vi "S8300E_CheckSN_Manual.vi"() -> ()   [LabVIEW 2011]
panel:
  out "UUT SN":string
  out "UUT MAC List":string
  out "CMD-LIST":cluster{string, string, string, string}[](array[cluster])
  out "log msg":string
  out "VISA resource name out":refnum<visa-resource-name>
  out "BEGIN TIME":u32
  out "進行狀況":string
  # "Error Code:SN-BIOS\nError Code:SN-DMI"
  # "S8300E Program SN (接UART COM9)"
  # "2014-12-12"
  # "Step1:Get Serial Number from BIOS Flash\nStep2:Get Serial Number from DMI table"
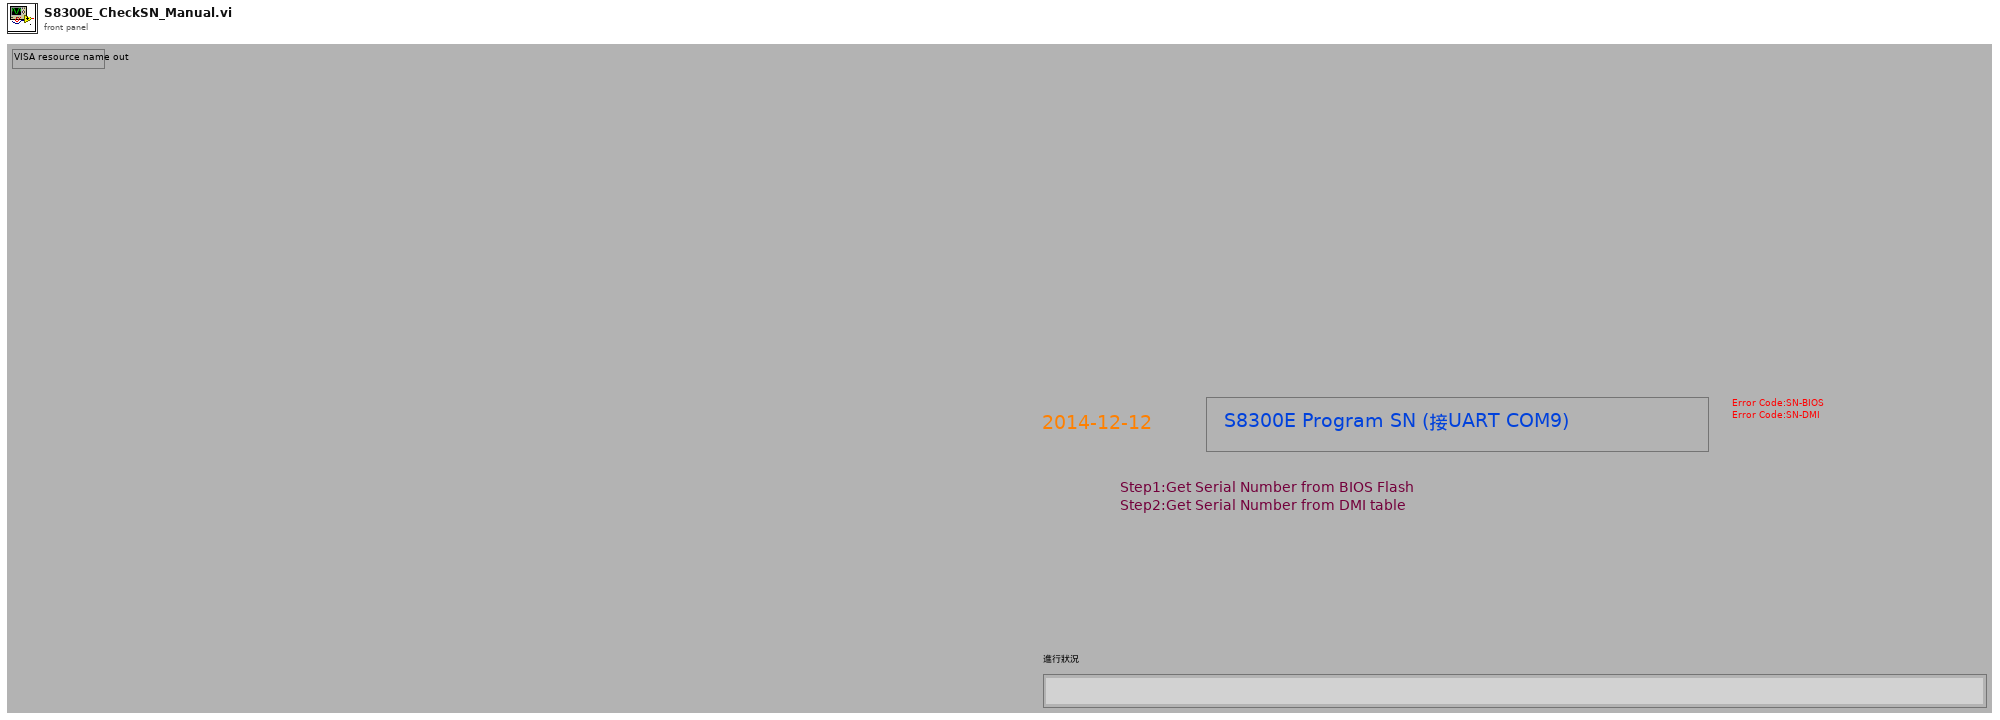
[diagram p1: front panel]
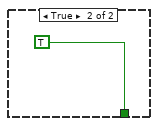
[diagram p7: hidden frame]
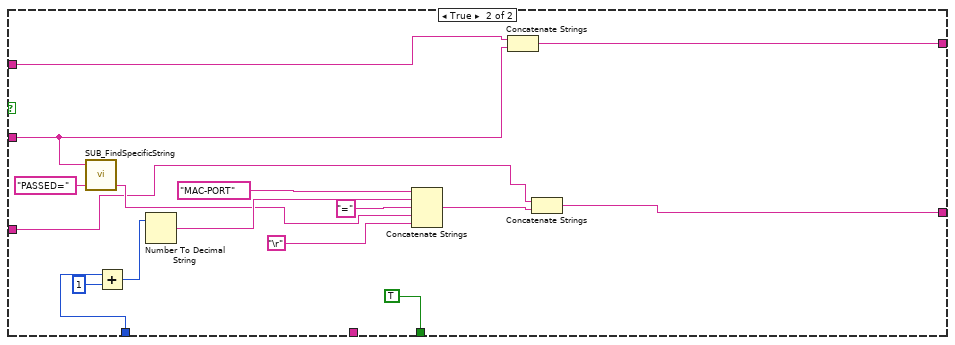
[diagram p9: hidden frame]
diagram:
  n1 = flat-sequence {
    frame #0 {
      n2 = Tick Count (ms)() -> (millisecond timer value=→"BEGIN TIME":u32)
    }
    frame #1 {
      n3 = property on="進行狀況" class="Str"("Blinking"=TRUE) -> ()  [unwired: 2 in, 2 out]
      "進行狀況" <- "進入測試準備中...." ("進行狀況")
      "UUT SN" <- ""
    }
    frame #2 {
      n4 = call "SUB_SearchFile_inFolder.vi"("Search Filename in Folder"="S8300E_sfcs_misc.txt") -> ("File Existing True/Flase"=w5:bool)  [unwired: 1 in]
      n5 = case shown="False" w5 {
        frame False {
          n6 = flat-sequence {
            frame #0 {
              n7 = call "Display Message to User"() -> ()  [unwired: 10 in, 2 out]
            }
            frame #1 {
              n8 = call "SUB_Writelog.vi"("Pass/Fail"="Fail:S8300E_CheckSN_Manual") -> ()  [unwired: 2 in]
            }
            frame #2 {
              n9 = Quit LabVIEW(quit? (T)=TRUE) -> ()
            }
          }
        }
        frame True {
        }
      }
    }
    frame #3 {
      n10 = call "Prompt User for Input"() -> ("待測物條碼序號"=w9:string)  [unwired: 17 in, 2 out]
      n11 = local write "UUT SN"(w9) -> ()
    }
    frame #4 {
      n12 = local read "UUT SN"() -> (w11:string)
      n13 = Concatenate Strings("PASSED=", w11) -> (w10:string)
      n14 = Concatenate Strings("PASSED=", w11) -> (w13:string)
      n15 = Concatenate Strings("./ser.sh -w -f  ", w11, "\r") -> (w32:string)
      n16 = Concatenate Strings("./ser.sh -r -f  ", "\r") -> (w28:string)
      n17 = Concatenate Strings("./ser.sh -r -d ", "\r") -> (w25:string)
      n18 = Bundle(w32, "PASSED=", "Set Serial Number to BIOS Flash", "SN-BIOS") -> ()  [unwired: 1 in, 1 out]
      n19 = Bundle(w28, w13, "Get Serial Number from BIOS Flash", "SN-BIOS") -> (w20:cluster{string, string, string, string})  [unwired: 1 in]
      n20 = Bundle(w25, w10, "Get Serial Number from DMI table", "SN-DMI") -> (w19:cluster{string, string, string, string})  [unwired: 1 in]
      n21 = Build Array(w20, w19) -> (→"CMD-LIST":cluster{string, string, string, string}[])
    }
    frame #5 {
      n22 = case shown="True" TRUE {
        frame False {
        }
        frame True {
          n23 = call "SUB_COM1_CLOSE.vi"("VISA resource name"=refnum<visa-resource-name> "COM9") -> ()  [unwired: 3 in]
        }
      }
    }
    frame #6 {
      n24 = case shown="True" TRUE {
        frame False {
        }
        frame True {
          n25 = call "SUB_COM9_INIT.vi"("baud rate"=u32 115200) -> ("VISA resource name out"=w40:refnum<visa-resource-name>)  [unwired: 1 in, 1 out]
          "VISA resource name out" <- w40
          n26 = call "SUB_COM1Wrt.vi"("VISA resource name"=w40, "write buffer"="\r") -> ("duplicate VISA resource name"=w37:refnum<visa-resource-name>)  [unwired: 1 in, 1 out]
          n27 = call "SUB_ContinueCom1Read.vi"("Numeric"=1200, "duplicate VISA resource name 2"=w37) -> ()  [unwired: 1 in, 3 out]
        }
      }
    }
    frame #7 {
      n28 = case shown="True" TRUE {
        frame False {
        }
        frame True {
          n29 = while {
            stop <- w52 stop-if-true
            w43 = "\r"
            n30 = Concatenate Strings(w43, w43, w43) -> (w44:string)
            n31 = local read "VISA resource name out"() -> (w45:refnum<visa-resource-name>)
            n32 = call "SUB_COM1Wrt.vi"("VISA resource name"=w45, "write buffer"=w44) -> ("duplicate VISA resource name"=w51:refnum<visa-resource-name>)  [unwired: 1 in, 1 out]
            n33 = Tick Count (ms)() -> (millisecond timer value=w50:u32)
            n34 = call "SUB_READ_COM1_FindString_timeout.vi"("Find this String"="s8300e_func_test#", "Timeout Seccond"=3.0, "Begin time"=w50, "duplicate VISA resource name 2"=w51) -> ("Output String"=w46:string, "Found String"=w47:bool)  [unwired: 1 in, 1 out]
            n35 = case shown="False" w47 {
              tunnel: [w54 TRUE] -> w52
              tunnel: w46 -> [w53 _]
              frame False {
                n36 = call "SUB_YESNO.vi"("Debug View"=w53, "Status"="UART無正確反應!需有S8300E字串") -> ("yes/no"=w57:enum32{"No Selection", "Yes", "No", "None"})  [unwired: 1 in]
                n37 = Equal?(x=w57, y=enum32{"No Selection", "Yes", "No", "None"}."No") -> (x = y?=w55:bool)
                n38 = case shown="True" w55 {
                  tunnel: [_ w59] -> w54
                  frame False {
                  }
                  frame True {
                    n39 = flat-sequence {
                      tunnel: [w63] -> w59
                      frame #0 {
                        n40 = call "SUB_Writelog.vi"("Pass/Fail"="Fail:S8300E_CheckSN_Manual") -> ()  [unwired: 2 in]
                      }
                      frame #1 {
                        n41 = call "SUB_SFCS_SendResult.vi"("ErrorCode"="UART", "PASS_Fail (1/0)"=i8 0) -> ()  [unwired: 1 out]
                      }
                      frame #2 {
                        w63 = TRUE ("quit? (T)")
                        n42 = Quit LabVIEW(quit? (T)=w63) -> ()
                      }
                    }
                  }
                }
              }
              frame True {
              }
            }
          }
        }
      }
    }
    frame #8 {
      n43 = local read "CMD-LIST"() -> (w67:cluster{string, string, string, string}[])
      n44 = Array Size(array=w67) -> (size(s)=w70:i32)
      n45 = for {
        N: w70 -> [_]
        shift-right: [w75] -> w68
        shift-left: "" -> [w74]
        shift-right: [w72] -> w65
        shift-left: "" -> [w71]
        i -> [w73]
        n46 = while {
          tunnel: w73 -> [w94]
          tunnel: [w86] -> w75
          tunnel: w74 -> [w85]
          tunnel: w73 -> [w78]
          tunnel: [w77] -> w72
          tunnel: w71 -> [w76]
          stop <- w88 stop-if-true
          n47 = local read "VISA resource name out"() -> (w90:refnum<visa-resource-name>)
          n48 = local read "CMD-LIST"() -> (w84:cluster{string, string, string, string}[])
          n49 = Index Array(array=w84, index=w94) -> (element=w83:cluster{string, string, string, string})
          n50 = Unbundle(w83) -> (w82:string, w80:string, w81:string, w79:string)
          n51 = call "SUB_COM1Wrt.vi"("VISA resource name"=w90, "write buffer"=w82) -> ("duplicate VISA resource name"=w93:refnum<visa-resource-name>)  [unwired: 1 in, 1 out]
          n52 = Tick Count (ms)() -> (millisecond timer value=w92:u32)
          n53 = call "SUB_READ_COM1_FindString_timeout.vi"("Find this String"=w80, "Timeout Seccond"=2.0, "Begin time"=w92, "duplicate VISA resource name 2"=w93) -> ("Output String"=w87:string, "Found String"=w89:bool)  [unwired: 1 in, 1 out]
          n54 = local write "進行狀況"(w81) -> ()
          n55 = case shown="False" w89 {
            tunnel: [_ TRUE] -> w88
            tunnel: w87 -> [w105 w122]
            tunnel: [w101 w127] -> w86
            tunnel: w85 -> [w101 w126]
            tunnel: w79 -> [w100 _]
            tunnel: w78 -> [_ w118]
            tunnel: [w95 w114] -> w77
            tunnel: w76 -> [w95 w113]
            frame False {
              n56 = local read "進行狀況"() -> (w97:string)
              n57 = Concatenate Strings("失敗!" ("string"), "\r", w97) -> (w96:string)
              n58 = call "SUB_YESNO.vi"("Debug View"=w105, "Status"=w96) -> ("yes/no"=w104:enum32{"No Selection", "Yes", "No", "None"})  [unwired: 1 in]
              n59 = Equal?(x=w104, y=enum32{"No Selection", "Yes", "No", "None"}."No") -> (x = y?=w102:bool)
              n60 = case shown="True" w102 {
                tunnel: w100 -> [_ w106]
                frame False {
                }
                frame True {
                  n61 = flat-sequence {
                    tunnel: [w108] -> w107
                    tunnel: w106 -> [w108]
                    tunnel: w107 -> [w110]
                    frame #0 {
                      n62 = call "SUB_Writelog.vi"("Pass/Fail"="Fail:S8300E_CheckSN_Manual") -> ()  [unwired: 2 in]
                    }
                    frame #1 {
                      n63 = call "SUB_SFCS_SendResult.vi"("ErrorCode"=w110, "PASS_Fail (1/0)"=i8 0) -> ()  [unwired: 1 out]
                    }
                    frame #2 {
                      n64 = Quit LabVIEW(quit? (T)=TRUE) -> ()
                    }
                  }
                }
              }
            }
            frame True {
              n65 = call "SUB_FindSpecificString.vi"("Find this String"="PASSED=", "String data"=w122) -> ("before \"; \" string"=w120:string)  [unwired: 2 in, 1 out]
              n66 = Add(x=w118, y=1) -> (x+y=w116:i32)
              n67 = Number To Decimal String(number=w116) -> (decimal integer string=w124:string)  [unwired: 1 in]
              n68 = Concatenate Strings("MAC-PORT" ("string"), w124, "=" ("string"), w120, "\r") -> (w115:string)
              n69 = Concatenate Strings(w126, w122) -> (w127:string)
              n70 = Concatenate Strings(w113, w115) -> (w114:string)
            }
          }
        }
      }
      "log msg" <- w68
      "UUT MAC List" <- w65
    }
    frame #9 {
      w132 = "\n"
      n71 = local read "log msg"() -> (w133:string)
      n72 = local read "UUT MAC List"() -> (w131:string)
      n73 = local read "BEGIN TIME"() -> (w137:u32)
      n74 = Tick Count (ms)() -> (millisecond timer value=w136:u32)
      n75 = call "SUB_CAL_TESTTIME.vi"("Test Item name"="S8300E_CheckSN_Manual", "Stop tick time"=w136, "Start tick time"=w137) -> ("Test Time output"=w130:string)  [unwired: 2 in]
      n76 = call "SUB_COM1_CLOSE.vi"("VISA resource name"=refnum<visa-resource-name> "COM9") -> ()  [unwired: 3 in]
      n77 = Concatenate Strings("Pass:S8300E_CheckSN_Manual", w132, w133, w132, w131, w130) -> (w135:string)
      n78 = call "SUB_Writelog.vi"("Pass/Fail"=w135) -> ()  [unwired: 2 in]
    }
    frame #10 {
      n79 = Request Deallocation(TRUE ("flag")) -> ()
    }
    frame #11 {
      n80 = Quit LabVIEW(quit? (T)=TRUE ("stop? (T)")) -> ()
    }
  }
